vi "AM_BJT_Char_Sweep.vi"(3 "error in (no error)":errorcluster, 4 "BJT Swp In":T2={"Vb / V"=0.0, "Vhi / V"=0.0, "Vlo / V"=0.0, "Vinc / V"=0.0, "Rb / kOhm"=0.0, "Rc / kOhm"=0.0, "Delay (ms)"=500, "Nreads"=3} {"Nreads" min=3 max=50 step=1; "Delay (ms)" min=4000 max=20000 step=1}, 5 "VISA resource name":refnum<visa-resource-name>) -> (0 "error out":errorcluster, 1 "SwpData":dbl[][](array[numeric]), 2 "VISA resource name 2":refnum<visa-resource-name>)   [LabVIEW 2018]
doc: "Sweep over Vc while Vb fixed to determine the IV characteristic of a BJT\n\nMeasurement (Raw Data):\nA0 = Vrc-hi, A1 = Vrc-lo, A2 = Vrb-hi, A3 = Vrb-lo, A4 = A1 = Vce, A5 = Gnd\n\nOutput (Formatted Data):\nVbin = A2, Vcin = A0, Irb = A2 - A3 / Rb, Irc = A0 - A1 / Rc, Vce = A4 - A5\n\nR. Sheehan 2 - 12 - 2020"
panel:
  in  "Meas Inputs":T1={"Vb / V"=0.0, "Vc / V"=0.0, "Rb / kOhm"=0.0, "Rc / kOhm"=0.0, "Delay (ms)"=500, "Nreads"=3} {"Nreads" min=3 max=50 step=1; "Delay (ms)" min=1000 max=20000 step=1}
  # "Measurement (Raw Data):\nA0 = Vrc-hi, A1 = Vrc-lo, A2 = Vrb-hi, A3 = Vrb-lo, A4 = A1 = Vce, A5 = Gnd\n\nOutput (Formatted Data):\nVbin = A2, Vcin = A0, Irb = A2 - A3 / Rb, Irc = A0 - A1 / Rc, Vce = A4 - A5"
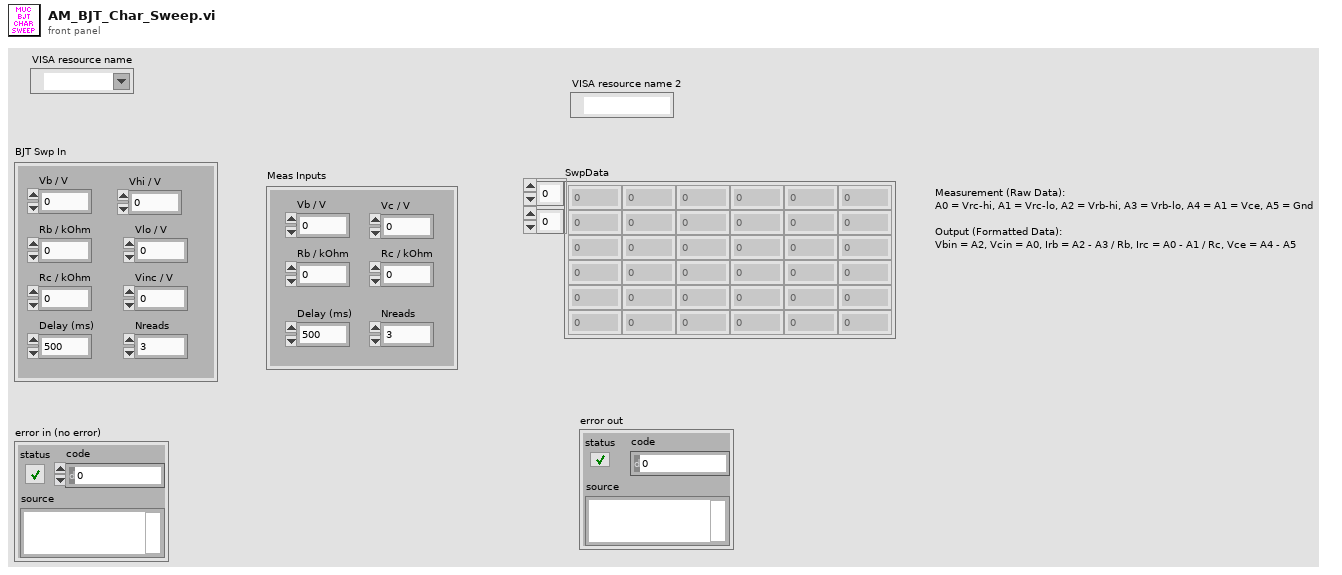
[diagram p1: front panel]
types:
  T1 = cluster{"Vb / V":dbl, "Vc / V":dbl, "Rb / kOhm":dbl, "Rc / kOhm":dbl, "Delay (ms)":u32, "Nreads":i32}
  T2 = cluster{"Vb / V":dbl, "Vhi / V":dbl, "Vlo / V":dbl, "Vinc / V":dbl, "Rb / kOhm":dbl, "Rc / kOhm":dbl, "Delay (ms)":u32, "Nreads":i32}
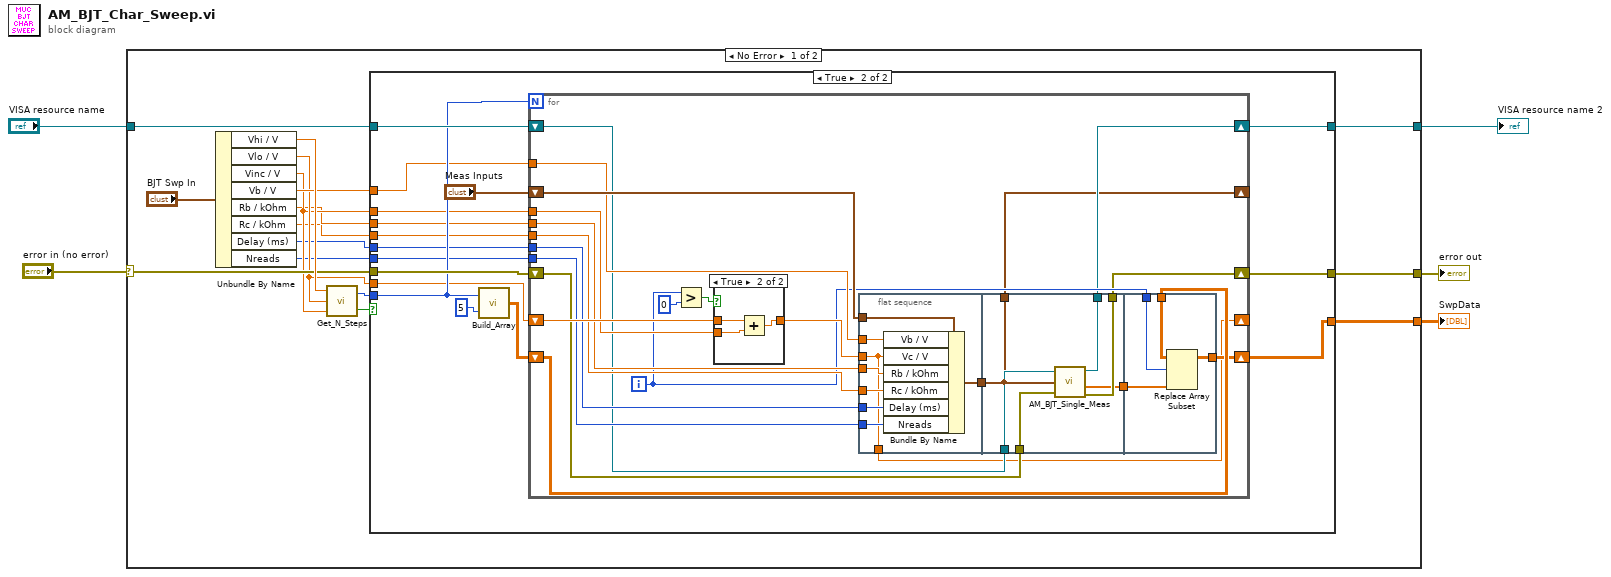
[diagram p0: block diagram]
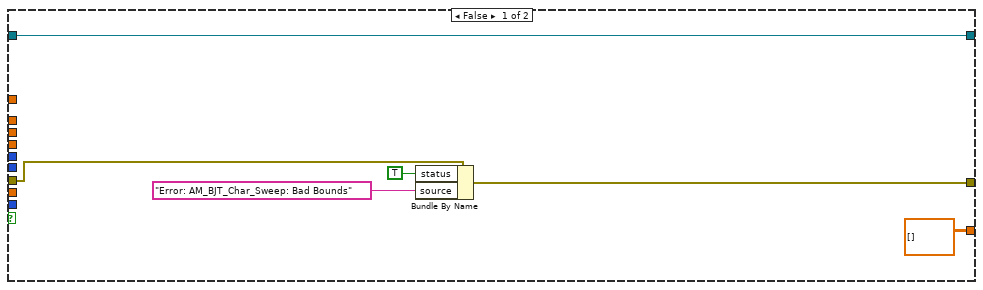
[diagram p2: hidden frame]
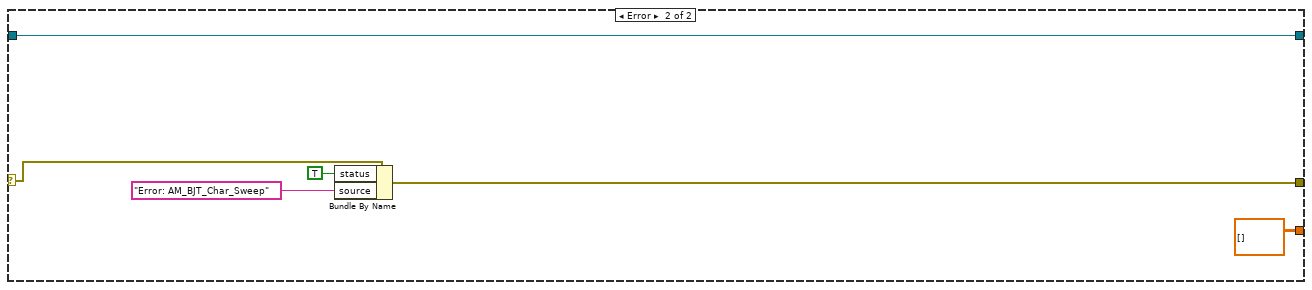
[diagram p4: hidden frame]
diagram:
  n1 = case shown="No Error" "error in (no error)" {
    selector: "error in (no error)" -> [w16 w93]
    tunnel: [w15 w92] -> w4
    tunnel: "VISA resource name" -> [w18 w91]
    tunnel: [w17 w91] -> w2
    tunnel: [w13 dbl[][] [] ("Array")] -> w1
    frame No Error {
      n2 = Unbundle By Name("BJT Swp In") -> ("Vhi / V"=w20:dbl, "Vlo / V"=w11:dbl, "Vinc / V"=w10:dbl, "Vb / V"=w12:dbl, "Rb / kOhm"=w9:dbl, "Rc / kOhm"=w8:dbl, "Delay (ms)"=w7:u32, "Nreads"=w6:i32)
      n3 = call "Get_N_Steps.vi"("Increment"=w10, "Lower Limit"=w11, "Upper Limit"=w20) -> ("Bounds Are Good"=w19:bool, "N steps"=w14:i32)
      n4 = case shown="True" w19 {
        tunnel: w18 -> [w27 w43]
        tunnel: [w27 w42] -> w17
        tunnel: w16 -> [w26 w41]
        tunnel: [w25 w40] -> w15
        tunnel: w14 -> [_ w39]
        tunnel: [dbl[][] [] ("Array") w36] -> w13
        tunnel: w12 -> [_ w34]
        tunnel: w11 -> [_ w33]
        tunnel: w10 -> [_ w32]
        tunnel: w9 -> [_ w31]
        tunnel: w8 -> [_ w30]
        tunnel: w7 -> [_ w29]
        tunnel: w6 -> [_ w28]
        frame False {
          n5 = Bundle By Name(cluster=w26, "status"=TRUE, "source"="Error: AM_BJT_Char_Sweep: Bad Bounds") -> (w25:errorcluster)
        }
        frame True {
          n6 = call "Build_Array.vi"("Ncolumns"=5, "Nrows"=w39) -> ("Array"=w37:dbl[][])
          n7 = for {
            N: w39 -> [_]
            shift-right: [w51] -> w42
            shift-left: w43 -> [w52]
            shift-right: [w49] -> w40
            shift-left: w41 -> [w50]
            shift-right: [w46] -> w36
            shift-left: w37 -> [w47]
            shift-right: [w48] -> _
            shift-left: "Meas Inputs" -> [w65]
            tunnel: w34 -> [w64]
            shift-right: [w44] -> _
            shift-left: w33 -> [w61]
            tunnel: w32 -> [w60]
            tunnel: w31 -> [w58]
            tunnel: w30 -> [w57]
            tunnel: w29 -> [w56]
            tunnel: w28 -> [w55]
            i -> [w53]
            n8 = Greater?(x=w53, y=0) -> (0:w62:bool)
            n9 = case shown="True" w62 {
              tunnel: w61 -> [w84 w87]
              tunnel: w60 -> [_ w86]
              tunnel: [w84 w85] -> w59
              frame False {
              }
              frame True {
                n10 = Add(x=w87, y=w86) -> (x+y=w85:dbl)
              }
            }
            n11 = flat-sequence {
              tunnel: w65 -> [w73]
              tunnel: w64 -> [w72]
              tunnel: w59 -> [w66]
              tunnel: w58 -> [w71]
              tunnel: w57 -> [w70]
              tunnel: w56 -> [w69]
              tunnel: w55 -> [w68]
              tunnel: [w67] -> w54
              tunnel: [w66] -> w44
              tunnel: w54 -> [w75]
              tunnel: w52 -> [w79]
              tunnel: [w78] -> w51
              tunnel: w50 -> [w77]
              tunnel: [w76] -> w49
              tunnel: [w75] -> w48
              tunnel: [w74] -> w45
              tunnel: w53 -> [w83]
              tunnel: w47 -> [w82]
              tunnel: [w81] -> w46
              tunnel: w45 -> [w80]
              frame #0 {
                n12 = Bundle By Name(cluster=w73, "Vb / V"=w72, "Vc / V"=w66, "Rb / kOhm"=w71, "Rc / kOhm"=w70, "Delay (ms)"=w69, "Nreads"=w68) -> (w67:T1)
              }
              frame #1 {
                n13 = call "AM_BJT_Single_Meas.vi"("VISA resource name"=w79, "Inputs"=w75, "error in (no error)"=w77) -> ("VISA resource name 2"=w78:refnum<visa-resource-name>, "Formatted Data"=w74:dbl[], "error out"=w76:errorcluster)  [unwired: 1 out]
              }
              frame #2 {
                n14 = Replace Array Subset(array=w82, new element=w80, index (row)=w83) -> (w81:dbl[][])  [unwired: 1 in]
              }
            }
          }
        }
      }
    }
    frame Error {
      n15 = Bundle By Name(cluster=w93, "status"=TRUE, "source"="Error: AM_BJT_Char_Sweep") -> (w92:errorcluster)
    }
  }
  "VISA resource name 2" <- w2
  "error out" <- w4
  "SwpData" <- w1
